vi "create queue.vi"(7 "max queue size (-1, unlimited)":i32=-1, 8 "error in (no error)":errorcluster, 9 "create if not found? (T)":bool=TRUE, 11 "name (unnamed)":string) -> (0 "error out":errorcluster, 1 "created new?":bool, 3 "queue out":refnum<queue>)   [LabVIEW 2025, in "ED Queued State Machine.lvlib"]
doc: "The type of data that the queue will host is defined. The data type is a cluster containing a string for the status and a variant for the data."
uses:
  ED Queued State Machine.lvlib
  state & data--cluster.ctl
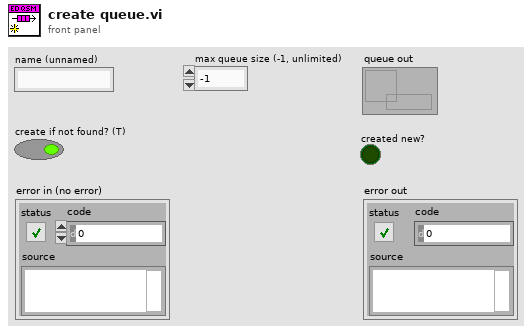
[diagram p1: front panel]
types:
  T1 = typedef "ED Queued State Machine.lvlib/state & data--cluster.ctl" = cluster{"State":string, "Data":variant}
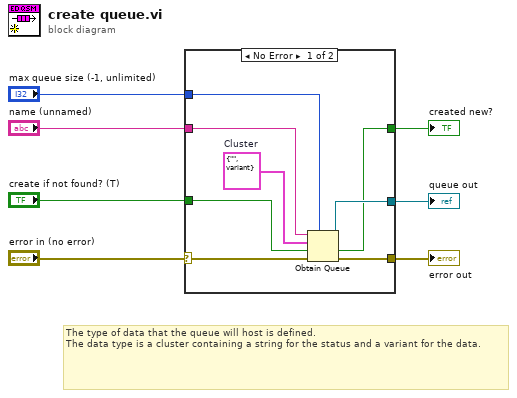
[diagram p0: block diagram]
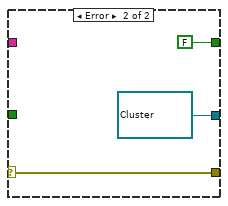
[diagram p2: hidden frame]
diagram:
  # "The type of data that the queue will host is defined. \nThe data type is a cluster containing a string for the status and a variant for the data."
  n1 = case shown="No Error" "error in (no error)" {
    selector: "error in (no error)" -> [w12 w18]
    tunnel: [w15 w18] -> w7
    tunnel: [w14 refnum<queue> refnum ("queue out")] -> w6
    tunnel: "name (unnamed)" -> [w11 _]
    tunnel: [w10 FALSE ("created new?")] -> w3
    tunnel: "max queue size (-1, unlimited)" -> [w9 _]
    tunnel: "create if not found? (T)" -> [w8 _]
    frame No Error {
      w13 = T1 {"State"="", "Data"=variant}  # Cluster
      n2 = Obtain Queue(max queue size (-1, unlimited)=w9, name (unnamed)=w11, element data type=w13, create if not found? (T)=w8, error in (no error)=w12) -> (queue out=w14:refnum<queue>, created new?=w10:bool, error out=w15:errorcluster)
    }
    frame Error {
    }
  }
  "error out" <- w7
  "queue out" <- w6
  "created new?" <- w3
